vi "Bundle.vi"(5 "Digit Resolution":T1=enum."5½", 6 "Target Measurement Count":i32=1, 7 "Range":dbl, 8 "error in (no error)":errorcluster, 9 "Function":T2, 10 "Measurements":dbl[](array[numeric]), 11 "DMM Measurement Data in":refnum<class "DMM Measurement Data.lvclass">) -> (0 "error out":errorcluster, 3 "DMM Measurement Data out":refnum<class "DMM Measurement Data.lvclass">)   [LabVIEW 2020, in "DMM Msg.lvlib" / "DMM Measurement Data.lvclass"]
doc: "Populate the data class."
uses:
  DMM Measurement Data.lvclass
  PPL/HDH.Driver.DMM.lvlibp/Controls/Ctl_Function.ctl
  PPL/HDH.Driver.DMM.lvlibp/Controls/Ctl_DigitResolution.ctl
  DMM Measurement Data.lvclass/DMM Measurement Data.ctl
  PPL/HDH.Driver.DMM.lvlibp
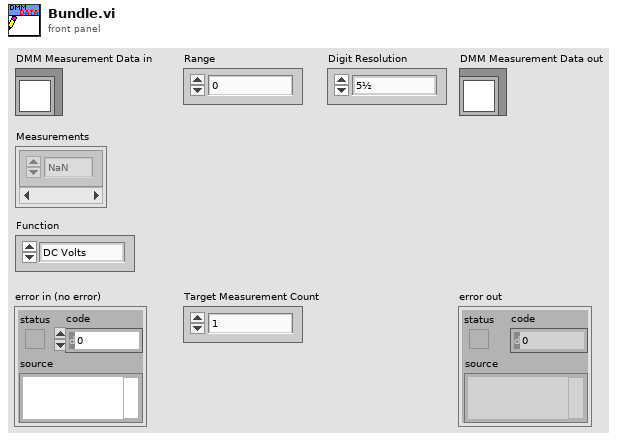
[diagram p1: front panel]
types:
  T1 = typedef "HDH.Driver.DMM.lvlibp/Ctl_DigitResolution.ctl" = enum8{"3½", "4½", "5½", "6½", "7½"}
  T2 = typedef "HDH.Driver.DMM.lvlibp/Ctl_Function.ctl" = enum8{"DC Volts", "AC Volts", "DC Current", "AC Current", "2-wire Resistance", "4-wire Resistance", "Diode", "Frequency", "Period", "AC Volts DC Coupled", "Capacitance", "Inductance", "Temperature"}
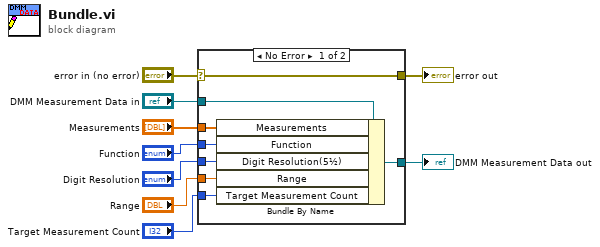
[diagram p0: block diagram]
diagram:
  n1 = case shown="No Error" "error in (no error)" {
    selector: "error in (no error)" -> [w17 w18]
    tunnel: [w17 w18] -> w8
    tunnel: [w15 w19] -> w6
    tunnel: "DMM Measurement Data in" -> [w16 w19]
    tunnel: "Measurements" -> [w14 _]
    tunnel: "Function" -> [w13 _]
    tunnel: "Digit Resolution" -> [w12 _]
    tunnel: "Range" -> [w11 _]
    tunnel: "Target Measurement Count" -> [w10 _]
    frame No Error {
      n2 = Bundle By Name(cluster=w16, "Measurements"=w14, "Function"=w13, "Digit Resolution(5½)"=w12, "Range"=w11, "Target Measurement Count"=w10) -> (w15:refnum<class "DMM Measurement Data.lvclass">)
    }
    frame Error {
    }
  }
  "error out" <- w8
  "DMM Measurement Data out" <- w6
